vi "Stop Module.vi"(6 "Timeout to Wait for Stop (s) (-1: no timeout)":dbl=-1.0, 8 "error in (no error)":errorcluster, 9 "Wait for Module to stop? (F)":bool, 10 "Origin":string) -> (0 "error out":errorcluster)   [LabVIEW 2015, in "TestStand Manager_DQMH.lvlib"]
doc: "Send the Stop request to the Module's Main.vi.\n_____\nBased on Delacor QMH Project Template 2.0.0.62.\n\nIf <b>Wait for Module to Stop?</b> is TRUE, this VI will wait until the module main VI stops, and will timeout at the <b>Timeout to Wait for Stop</b> value. This value defaults to \"-1\", which means the VI will not timeout, and will always wait until the module main VI stops before completing execution.\n\nNote: The <b>Timeout to Wait for Stop</b> value is ignored if 'Wait for Module to Stop?' is set to FALSE.\n\n<b>Note:</b> This VI was modified by the <b>Validate DQMH Module</b> tool to upgrade it to the DQMH 2.1 approach to stopping a singleton module.\n____\nDelacor QMH Thermal Chamber Examples 4.0.0.21\nCopyright (c) 2018, Delacor"
uses:
  TestStand Manager_DQMH.lvlib
  Stop Argument--cluster.ctl
  <vilib>/event_ctls.llb/usereventprio.ctl
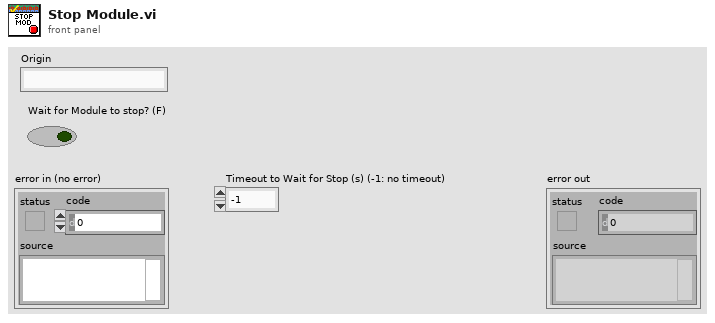
[diagram p1: front panel]
types:
  T1 = typedef "TestStand Manager_DQMH.lvlib/Stop Argument--cluster.ctl" = cluster{"Origin":string, "Exit via Stop Module Req?":bool, "Wait for Module to stop?":bool}
  T2 = typedef "usereventprio.ctl" = enum32{"high priority", "normal priority"}
  T3 = typedef "TestStand Manager_DQMH.lvlib/Request Events--cluster.ctl" = cluster{"Stop Module":refnum<user-event>, "Show Panel":refnum<user-event>, "Hide Panel":refnum<user-event>, "Get Module Execution Status":refnum<user-event>, "Show Diagram":refnum<user-event>}
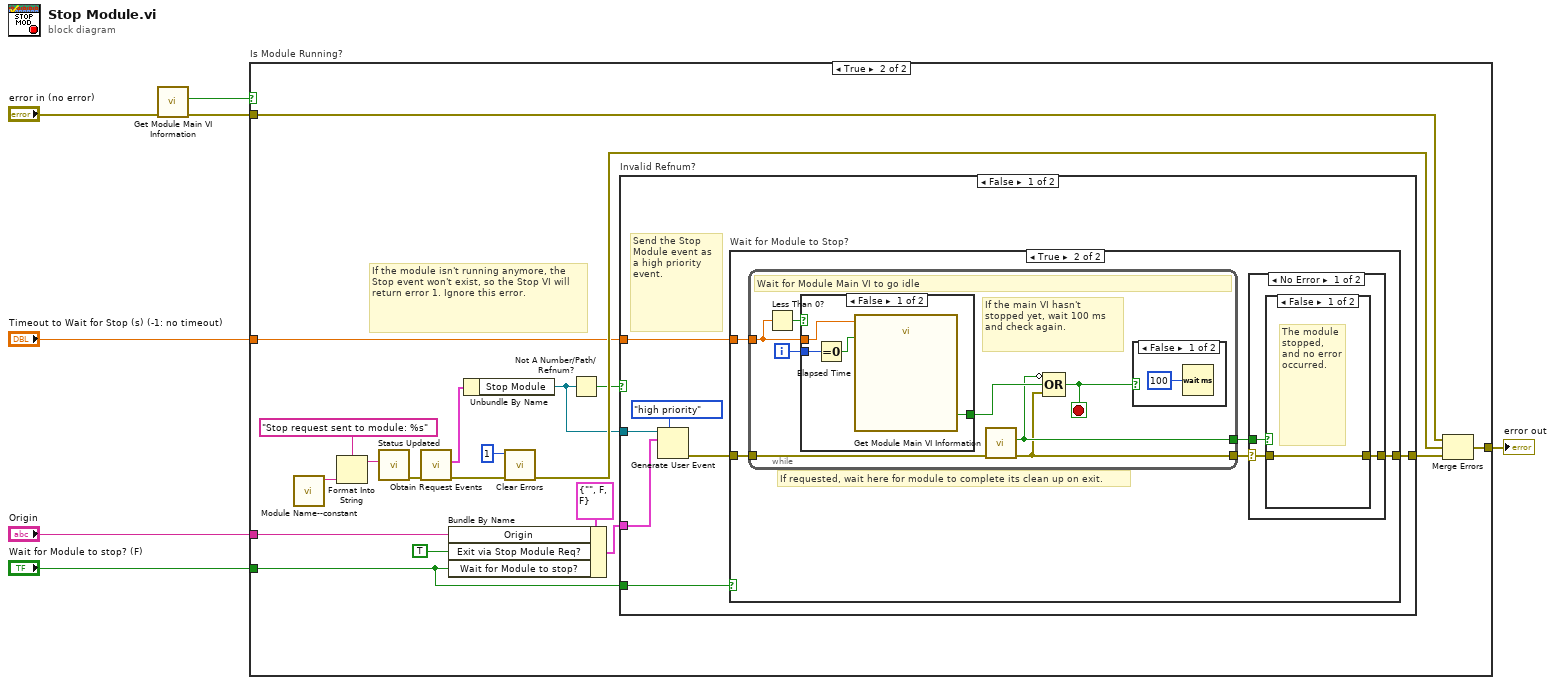
[diagram p0: block diagram]
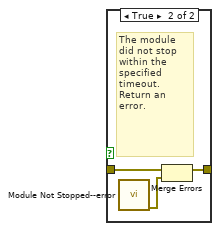
[diagram p4: hidden frame]
diagram:
  n1 = call "Get Module Main VI Information.vi"("error in (no error)"="error in (no error)") -> ("error out"=w5:errorcluster, "Is Module Running?"=w1:bool)  [unwired: 7 in, 2 out]
  n2 = case "Is Module Running?" shown="True" w1 {
    tunnel: [w8 w27] -> w7
    tunnel: "Origin" -> [_ w21]
    tunnel: w5 -> [w8 w25]
    tunnel: "Wait for Module to stop? (F)" -> [_ w13]
    tunnel: "Timeout to Wait for Stop (s) (-1: no timeout)" -> [_ w12]
    frame False {
      # "The module is not running, there is no need to run the Stop Module code."
    }
    frame True {
      # "If the module isn't running anymore, the Stop event won't exist, so the Stop VI will return error 1. Ignore this error."
      n3 = call "Module Name--constant.vi"() -> ("Module Name"=w11:string)  [unwired: 11 in]
      n4 = Format Into String(format string="Stop request sent to module: %s", w11) -> (resulting string=w10:string)  [unwired: 2 in, 1 out]
      n5 = call "Status Updated.vi"("Status"=w10) -> ("error out"=w23:errorcluster)  [unwired: 10 in]
      n6 = call "Obtain Request Events.vi"("error in (no error)"=w23) -> ("error out"=w22:errorcluster, "TestStand Manager_DQMH Request Events"=w9:T3)  [unwired: 9 in]
      n7 = Bundle By Name(cluster=T1 {"Origin"="", "Exit via Stop Module Req?"=FALSE, "Wait for Module to stop?"=FALSE} ("Stop Argument"), "Origin"=w21, "Exit via Stop Module Req?"=TRUE, "Wait for Module to stop?"=w13) -> (w16:T1)
      n8 = Unbundle By Name(w9) -> ("Stop Module"=w17:refnum<user-event>)
      n9 = call <vilib>:"Clear Errors.vi"("error in (no error)"=w22, "specific error code to clear (0: all)"=1) -> ("error out"=w24:errorcluster)  [unwired: 4 in, 1 out]
      n10 = Not A Number/Path/Refnum?(number/path/refnum=w17) -> (NaN/Path/Refnum?=w18:bool)
      n11 = case "Invalid Refnum?" shown="False" w18 {
        tunnel: [w33 _] -> w26
        tunnel: w17 -> [w32 _]
        tunnel: w16 -> [w30 _]
        tunnel: w13 -> [w29 _]
        tunnel: w12 -> [w28 _]
        frame False {
          # "Send the Stop Module event as a high priority event."
          n12 = Generate User Event(priority (normal)=usereventprio."high priority", user event=w32, event data cluster=w30) -> (error out=w34:errorcluster)  [unwired: 1 in, 1 out]
          n13 = case "Wait for Module to Stop?" shown="True" w29 {
            tunnel: w34 -> [w35 w40]
            tunnel: [w35 w38] -> w33
            tunnel: w28 -> [_ w37]
            frame False {
            }
            frame True {
              # "If requested, wait here for module to complete its clean up on exit."
              n14 = while {
                tunnel: w37 -> [w53]
                tunnel: w40 -> [w56]
                tunnel: [w49] -> w39
                tunnel: [w50] -> w36
                i -> [w55]
                stop <- w51 stop-if-true
                # "If the main VI hasn't stopped yet, wait 100 ms and check again."
                # "Wait for Module Main VI to go idle"
                n15 = Less Than 0?(x=w53) -> (x < 0?=w52:bool)
                n16 = case shown="False" w52 {
                  tunnel: w53 -> [w58 _]
                  tunnel: w55 -> [w60 _]
                  tunnel: [w59 _] -> w54
                  frame False {
                    n17 = Equal To 0?(x=w60) -> (x = 0?=w61:bool)
                    n18 = call "Elapsed Time"("Time Target (s)"=w58, "Reset"=w61) -> ("Time has Elapsed"=w59:bool)  [unwired: 10 in, 7 out]
                  }
                  frame True {
                    # "User specified a timeout of -1, so don't keep track of the elapsed time since this loop started."
                  }
                }
                n19 = call "Get Module Main VI Information.vi"("error in (no error)"=w56) -> ("error out"=w49:errorcluster, "Is Module Running?"=w50:bool)  [unwired: 7 in, 2 out]
                n20 = Compound Arithmetic op=OR(invert w50, w54, w49) -> (w51:bool)
                n21 = case shown="False" w51 {
                  frame False {
                    n22 = Wait (ms)(milliseconds to wait=u32 100) -> ()  [unwired: 1 out]
                  }
                  frame True {
                  }
                }
              }
              n23 = case shown="No Error" w39 {
                selector: w39 -> [w43 w48]
                tunnel: [w42 w48] -> w38
                tunnel: w36 -> [w41 _]
                frame No Error {
                  n24 = case shown="False" w41 {
                    tunnel: w43 -> [w44 w47]
                    tunnel: [w44 w46] -> w42
                    frame False {
                      # "The module stopped, and no error occurred."
                    }
                    frame True {
                      # "The module did not stop within the specified timeout. Return an error."
                      n25 = call "Module Not Stopped--error.vi"() -> ("error out"=w45:errorcluster)  [unwired: 11 in]
                      n26 = Merge Errors(w47, w45) -> (w46:errorcluster)
                    }
                  }
                }
                frame Error {
                  # "An error occurred while waiting for the module to stop. Return that error."
                }
              }
            }
          }
        }
        frame True {
          # "Module is exiting. No need to send the standard \"not running\" error that is sent in other request VIs."
        }
      }
      n27 = Merge Errors(w25, w24, w26) -> (w27:errorcluster)
    }
  }
  "error out" <- w7
